vi "Flatten Value.vi"(8 "error in (no error)":errorcluster, 11 "Boolean in":refnum<class "String.lvclass">) -> (0 "error out":errorcluster, 2 "Value":string, 3 "Boolean out":refnum<class "String.lvclass">)   [LabVIEW 2020, in "String.lvclass"]
uses:
  <vilib>/gpm_packages/@cs/data-type-serializer/source/String/String.lvclass
  <vilib>/gpm_packages/@cs/data-type-serializer/source/String/String.lvclass/String.ctl
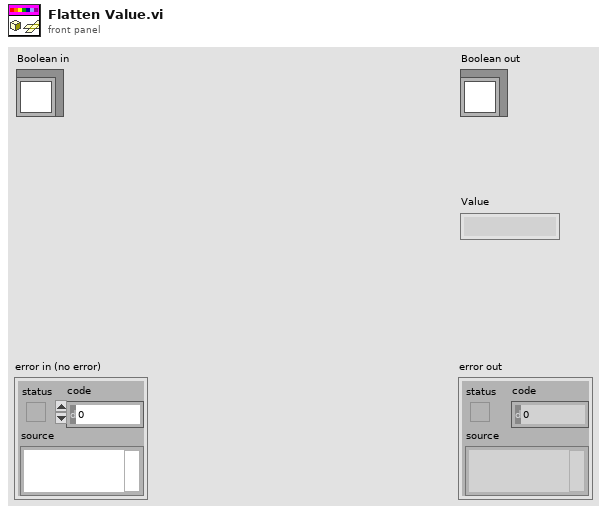
[diagram p1: front panel]
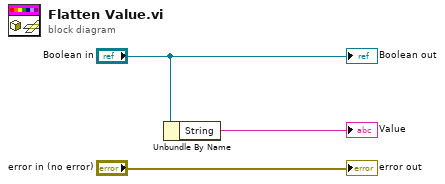
[diagram p0: block diagram]
diagram:
  n1 = Unbundle By Name("Boolean in") -> ("String"=→"Value":string)
  "error out" <- "error in (no error)"
  "Boolean out" <- "Boolean in"
